vi "modifyAnimate.vi"(8 "error in (no error)":errorcluster, 10 "Animate":bool, 11 "Filled Text Fields Actor in":refnum<class "Filled Text Fields Actor.lvclass">) -> (0 "error out":errorcluster, 3 "Filled Text Fields Actor out":refnum<class "Filled Text Fields Actor.lvclass">)   [LabVIEW 2017, in "Filled Text Fields Actor.lvlib" / "Filled Text Fields Actor.lvclass"]
uses:
  Filled Text Fields Actor.lvclass
  Filled Text Fields Actor.lvclass/Filled Text Fields Actor.ctl
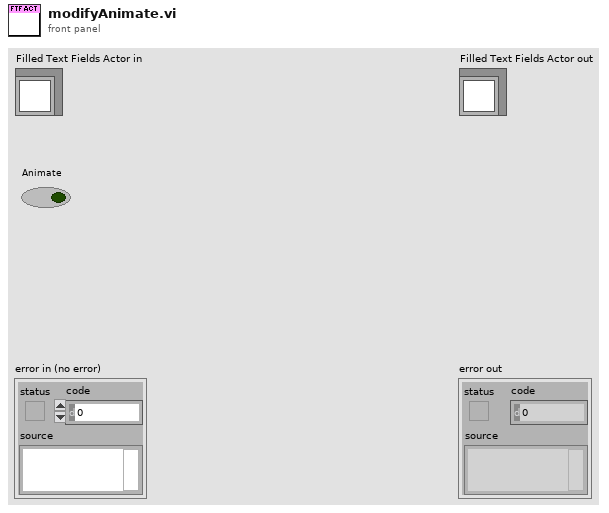
[diagram p1: front panel]
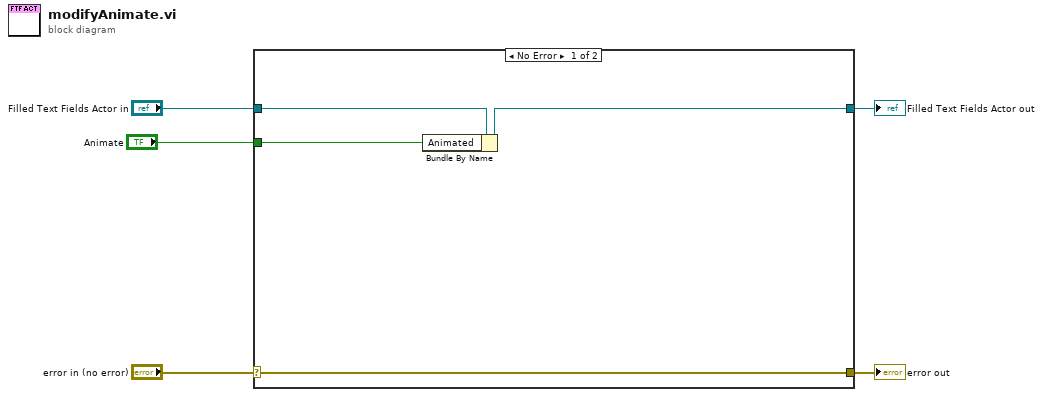
[diagram p0: block diagram]
diagram:
  n1 = case shown="No Error" "error in (no error)" {
    selector: "error in (no error)" -> [w8 w11]
    tunnel: [w8 w11] -> w4
    tunnel: [w7 w10] -> w2
    tunnel: "Filled Text Fields Actor in" -> [w9 w10]
    tunnel: "Animate" -> [w6 _]
    frame No Error {
      n2 = Bundle By Name(cluster=w9, "Animated"=w6) -> (w7:refnum<class "Filled Text Fields Actor.lvclass">)
    }
    frame Error {
    }
  }
  "error out" <- w4
  "Filled Text Fields Actor out" <- w2
